vi "EditorSub createPictureSelector.vi"   [LabVIEW 2018]
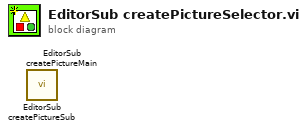
[diagram p0: block diagram]
diagram:
  n1 = call "EditorSub createPictureSub.vi"() -> ()  [unwired: 10 in, 2 out]
  n2 = call "EditorSub createPictureMain.vi"() -> ()  [unwired: 10 in, 2 out]
